vi "Unpack Tree Edit Cell.vi"(11 "TreeEditCellMsg":refnum<class "TreeEditCellMsg.lvclass">) -> (0 "String":string, 1 "Time":u32, 2 "Control Label":string, 3 "CtlRef":refnum<vi>, 4 "Tag":string, 6 "Col":i32)   [LabVIEW 2018, in "MVA Framework.lvlib" / "ActorEvents.lvlib" / "TreeEditCellMsg.lvclass"]
doc: "<License>\nCopyright © 2017 Composed Systems, LLC | All rights reserved\nwww.composed.io\n\nAuthor: Ethan Stern <ethan.stern@composed.io>\n\nThis software is provided \"AS IS\" WITHOUT WARRANTIES, either express or implied, AND IS FOR EDUCATIONAL PURPOSES ONLY.\n</License>"
uses:
  TreeEditCellMsg.lvclass
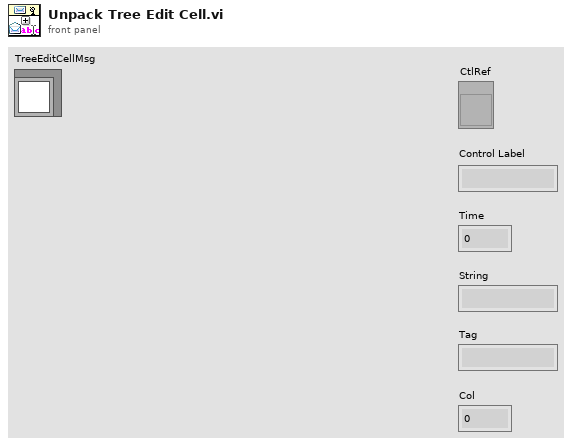
[diagram p1: front panel]
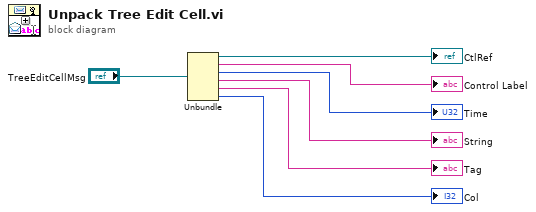
[diagram p0: block diagram]
diagram:
  n1 = Unbundle("TreeEditCellMsg") -> (→"CtlRef":refnum<vi>, →"Control Label":string, →"Time":u32, →"String":string, →"Tag":string, →"Col":i32)
